vi "Init Testbox.vi"(11 "MulticolumnListbox in":refnum<vi>) -> (3 "MulticolumnListbox in":refnum<vi>)   [LabVIEW 2013]
uses:
  <vilib>/Utility/miscctls.llb/LVRowAndColumnTypeDef.ctl
  <vilib>/Utility/miscctls.llb/LVRowAndColumnUnsignedTypeDef.ctl
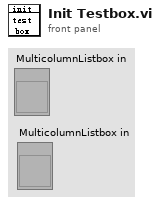
[diagram p1: front panel]
types:
  T1 = typedef "LVRowAndColumnUnsignedTypeDef.ctl" = cluster{"Row":u32, "Column":u32}
  T2 = typedef "LVRowAndColumnTypeDef.ctl" = cluster{"Row":i32, "Column":i32}
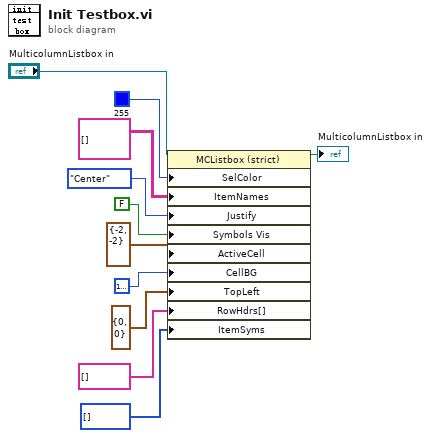
[diagram p0: block diagram]
diagram:
  n1 = property on="Property Node" class="MCListbox (strict)"(reference="MulticolumnListbox in", "SelColor"=u32 255, "ItemNames"=string[][] [] ("Item Names"), "Justify"=enum16{"Left", "Center", "Right"}."Center" ("Active Cell:Cell Justification"), "Symbols Vis"=FALSE ("Visible Items:Symbols Visible"), "ActiveCell"=T2 {"Row"=-2, "Column"=-2} ("Active Cell:Active Cell"), "CellBG"=u32 16777238, "TopLeft"=T1 {"Row"=0, "Column"=0} ("Top Left Visible Cell"), "RowHdrs[]"=string[] [] ("Row Header Strings[]"), "ItemSyms"=i32[] [] ("Item Symbols")) -> (reference out=→"MulticolumnListbox in":refnum<vi>)  [unwired: 1 in, 1 out]
